vi "Generate Lockin Comments.vi"(7 "error in (no error)":errorcluster, 9 "Channels: AO":T1={"AO amp (V)"=[0.01, 0.0, 0.0, 0.0, 0.0, 0.0, 0.0, 0.0], "AO DC (V)"=[0.0, 0.0, 0.0, 0.0, 0.0, 0.0, 0.0, 0.0], "AO f (Hz)"=[13.1, 13.0, 13.0, 13.0, 13.0, 13.0, 13.0, 13.0], "AO phi (°)"=[0.0, 0.0, 0.0, 0.0, 0.0, 0.0, 0.0, 0.0], "function"=[], "I+"=[]} {"AO f (Hz)" min=0.001 max=10000.0; "AO DC (V)" format="%.3p"; "AO amp (V)" format="%.3p"}, 10 "Comments in":string) -> (0 "error out":errorcluster, 3 "Comments":string)   [LabVIEW 2016, in "Control Experiment.lvclass"]
uses:
  Control Experiment.lvclass
  <userlib>/LevyLab/Lockin-Multichannel/Typedefs/AO-cluster.ctl
  <userlib>/LevyLab/Lockin-Multichannel/Typedefs/AO_Amp-array.ctl
  <userlib>/LevyLab/Lockin-Multichannel/Typedefs/AO_DC-array.ctl
  <userlib>/LevyLab/Lockin-Multichannel/Typedefs/AO_f-array.ctl
  <userlib>/LevyLab/Lockin-Multichannel/Typedefs/AO_phi-array.ctl
  <userlib>/LevyLab/Lockin-Multichannel/Typedefs/Function-array.ctl
  <userlib>/LevyLab/Lockin-Multichannel/Typedefs/Function-enum.ctl
panel:
  # "1"
  # "2"
  # "3"
  # "4"
  # "5"
  # "6"
  # "7"
  # "8"
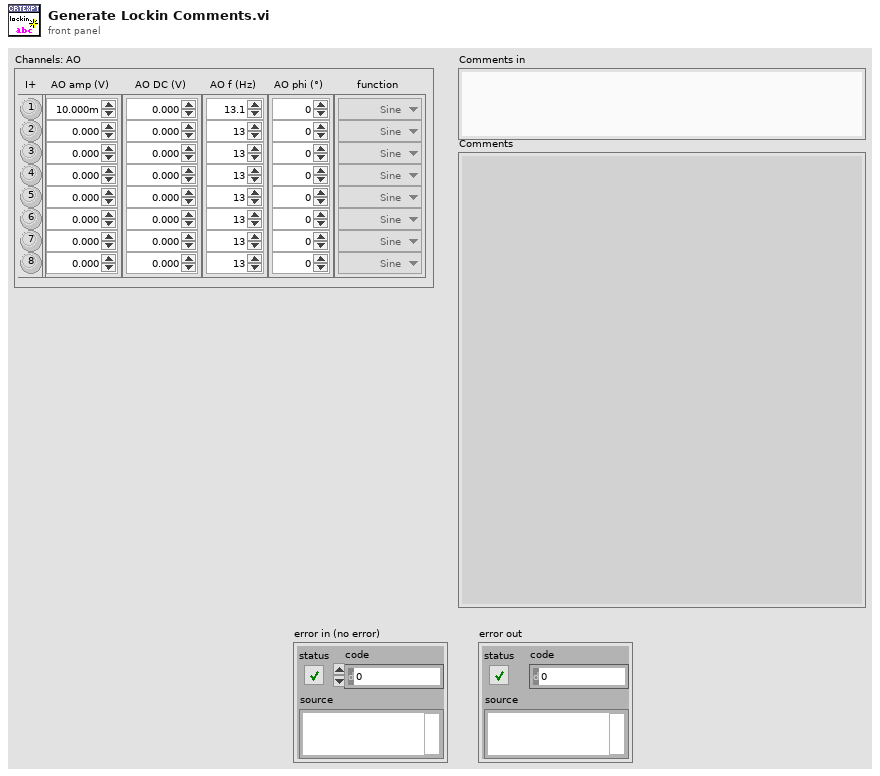
[diagram p1: front panel]
types:
  T1 = typedef "AO-cluster.ctl" = cluster{"AO amp (V)":T2, "AO DC (V)":T3, "AO f (Hz)":T4, "AO phi (°)":T5, "function":T6, "I+":bool[]}
  T2 = typedef "AO_Amp-array.ctl" = dbl[]
  T3 = typedef "AO_DC-array.ctl" = dbl[]
  T4 = typedef "AO_f-array.ctl" = dbl[]
  T5 = typedef "AO_phi-array.ctl" = dbl[]
  T6 = typedef "Function-array.ctl" = T7[]
  T7 = typedef "Function-enum.ctl" = enum16{"Sine", "Triangle", "Square", "Sawtooth"}
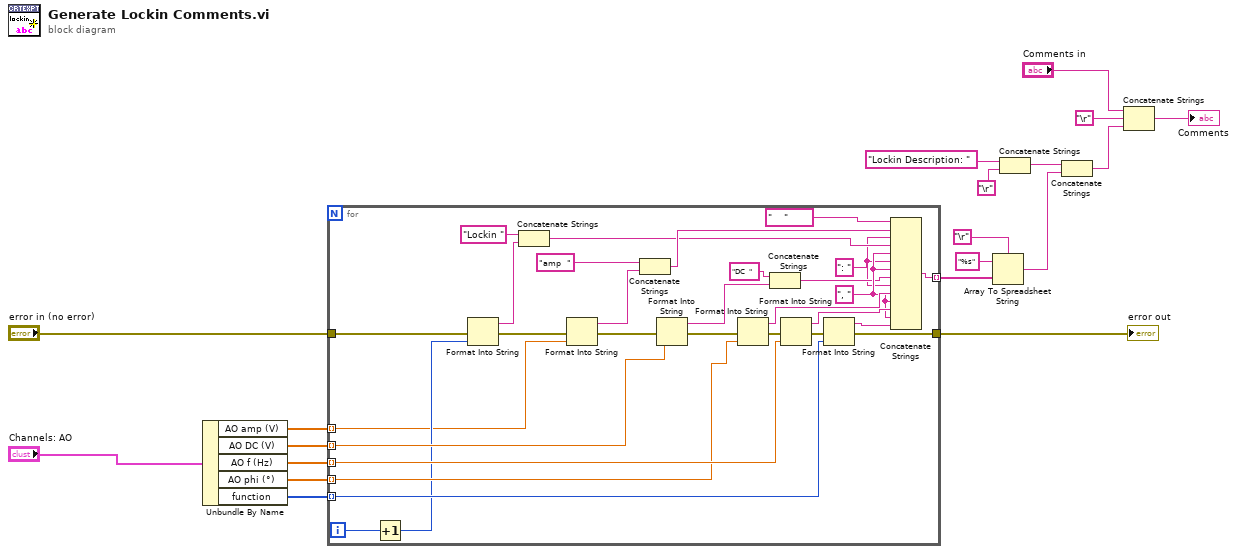
[diagram p0: block diagram]
diagram:
  n1 = Unbundle By Name("Channels: AO") -> ("AO amp (V)"=w15:T2, "AO DC (V)"=w16:T3, "AO f (Hz)"=w17:T4, "AO phi (°)"=w18:T5, "function"=w19:T6)
  n2 = for {
    tunnel: w15 -> [w21] mode=indexing
    tunnel: w16 -> [w35] mode=indexing
    tunnel: w17 -> [w45] mode=indexing
    tunnel: w18 -> [w44] mode=indexing
    tunnel: w19 -> [w39] mode=indexing
    tunnel: [w46] -> w10 mode=indexing
    tunnel: "error in (no error)" -> [w34]
    tunnel: [w29] -> w9
    i -> [w25]
    w41 = ", "
    w20 = ": "
    n3 = Increment(x=w25) -> (x+1=w24:i32)
    n4 = Format Into String(error in=w34, w24) -> (resulting string=w48:string, error out=w33:errorcluster)  [unwired: 2 in]
    n5 = Concatenate Strings("Lockin ", w48) -> (w27:string)
    n6 = Format Into String(error in=w33, w21) -> (resulting string=w23:string, error out=w26:errorcluster)  [unwired: 2 in]
    n7 = Concatenate Strings("amp  ", w23) -> (w28:string)
    n8 = Format Into String(error in=w26, w35) -> (resulting string=w36:string, error out=w32:errorcluster)  [unwired: 2 in]
    n9 = Format Into String(error in=w32, w44) -> (resulting string=w43:string, error out=w31:errorcluster)  [unwired: 2 in]
    n10 = Concatenate Strings("DC  ", w36) -> (w37:string)
    n11 = Format Into String(error in=w31, w45) -> (resulting string=w42:string, error out=w30:errorcluster)  [unwired: 2 in]
    n12 = Format Into String(error in=w30, w39) -> (resulting string=w40:string, error out=w29:errorcluster)  [unwired: 2 in]
    n13 = Concatenate Strings("    " ("string"), w28, w20, w27, w41, w20, w41, w37, w20, w43, w41, w42, w41, w40) -> (w46:string)
  }
  "error out" <- w9
  n14 = Array To Spreadsheet String(delimiter (Tab)="\r", array=w10, 3:"%s" ("format string")) -> (spreadsheet string=w5:string)
  n15 = Concatenate Strings("Lockin Description: " ("string"), "\r") -> (w6:string)
  n16 = Concatenate Strings(w6, w5) -> (w4:string)
  n17 = Concatenate Strings("Comments in", "\r", w4) -> (→"Comments":string)
